vi "Is Nominal State.vi"(11 "jettl Actor in":refnum<class "jettl Actor.lvclass">) -> (2 "Is Nominal State?":bool)   [LabVIEW 2021, in "jettl.lvlib" / "Temporary Actor.lvlib" / "jettl Actor.lvclass"]
uses:
  jettl Actor.lvclass
  State.ctl
  jettl Actor.lvclass/jettl Actor.ctl
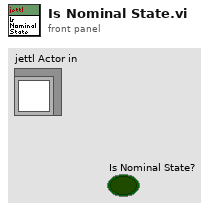
[diagram p1: front panel]
types:
  T1 = typedef "jettl.lvlib/Temporary Actor.lvlib/jettl Actor.lvclass/State.ctl" = enum16{"Nominal", "Teardown", "Error"}
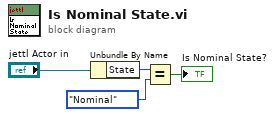
[diagram p0: block diagram]
diagram:
  n1 = Unbundle By Name("jettl Actor in") -> ("State"=w2:T1)
  n2 = Equal?(x=w2, y=State."Nominal") -> (x = y?=→"Is Nominal State?":bool)
